vi "To Text.vi"(3 "SPL":dbl, 4 "Ending Airflow":dbl, 5 "Starting Airflow":dbl, 6 "selected path":path, 7 "Header":string, 8 "error in (no error)":errorcluster, 9 "SGP":dbl, 10 "Resistance":dbl, 11 "Time":dbl) -> (0 "error out":errorcluster, 2 "resulting string":string)   [LabVIEW 2013]
panel:
  out "Trial":string
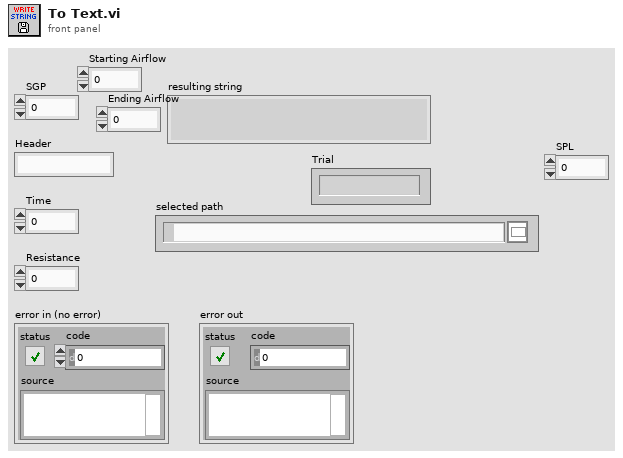
[diagram p1: front panel]
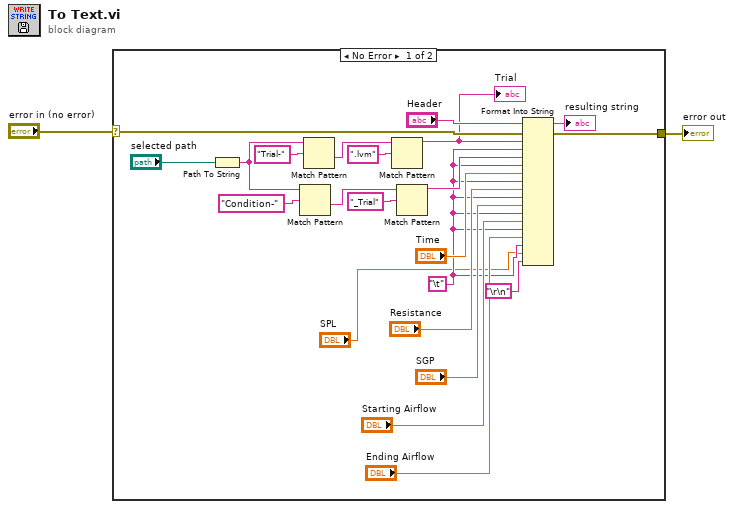
[diagram p0: block diagram]
diagram:
  n1 = case shown="No Error" "error in (no error)" {
    selector: "error in (no error)" -> [w22 w25]
    tunnel: [w21 w25] -> w1
    frame No Error {
      w4 = "\t"
      n2 = Path To String(path="selected path") -> (string=w18:string)
      n3 = Match Pattern(string=w18, regular expression="Condition-") -> (after substring=w16:string)  [unwired: 1 in, 3 out]
      n4 = Match Pattern(string=w18, regular expression="Trial-") -> (after substring=w8:string)  [unwired: 1 in, 3 out]
      n5 = Match Pattern(string=w8, regular expression=".lvm") -> (before substring=w6:string)  [unwired: 1 in, 3 out]
      "Trial" <- w6
      n6 = Match Pattern(string=w16, regular expression="_Trial") -> (before substring=w14:string)  [unwired: 1 in, 3 out]
      n7 = Format Into String(initial string="Header", error in=w22, w6, w4, w14, w4, "Time", w4, "Resistance", w4, "SGP", w4, "Starting Airflow", w4, "Ending Airflow", w4, "SPL", "\r\n") -> (resulting string=→"resulting string":string, error out=w21:errorcluster)  [unwired: 1 in]
    }
    frame Error {
    }
  }
  "error out" <- w1
